vi "LINX - Live reset.vi"() -> ()   [LabVIEW 2019]
uses:
  <vilib>/MakerHub/LINX/Public/Utilities/Open Serial.vi
  <vilib>/MakerHub/LINX/LMH-LINX.lvlib
  vi.lib/LINXx/LINXx.lvlib
panel:
  out "Connected?":bool
  in  "Reconnect wait time":u32=2000
  out "Loop Rate (Hz)":u32
  in  "stop":bool
  in  "Serial Port":refnum<visa-resource-name>="N/A"
  in  "Reset board":bool
  # "Setup"
  # "Status"
  # "Commands"
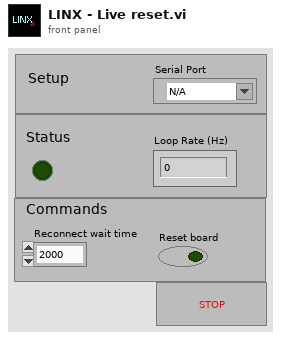
[diagram p1: front panel]
types:
  T1 = typedef "LMH-LINX.lvlib/LINX Ref.ctl" = cluster{"IO":T2, "Interface":T3, "LINX Device Config":T4}
  T2 = typedef "LMH-LINX.lvlib/Platform.ctl" = enum16{"Remote", "Local"}
  T3 = typedef "LMH-LINX.lvlib/Interface.ctl" = enum16{"Serial", "TCP"}
  T4 = typedef "LMH-LINX.lvlib/Device.lvlib/LINX Device Config.ctl" = cluster{"Interface":T3, "COM Port":refnum<visa-resource-name>, "TCP Configuration":T5, "Device Family":u8, "Device ID":u8, "Device Name":string, "TCP Ref":refnum<k5>, "Channels":T6}
  T5 = typedef "LMH-LINX.lvlib/Device.lvlib/TCP Config.ctl" = cluster{"IP Address":string, "Port":u16}
  T6 = typedef "LMH-LINX.lvlib/Channels.ctl" = cluster{"DI":u8[], "DO":u8[], "AI":u8[], "AO":u8[], "PWM":u8[], "QE":u8[], "UART":u8[], "I2C 2":u8[], "SPI":u8[], "CAN":u8[], "Servo":u8[], "AI Ref (V)":dbl, "AI Resolution (Bits)":u8, "AO Ref (V)":dbl, "AO Resolution (Bits)":u8}
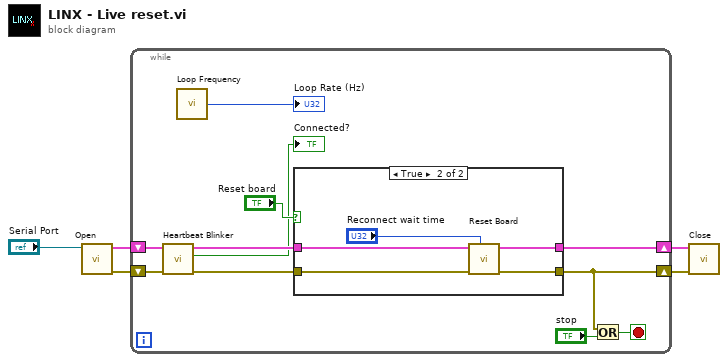
[diagram p0: block diagram]
diagram:
  n1 = call-poly <vilib>:"Open.vi"("Serial Port"="Serial Port") -> ("Error Out"=w4:errorcluster, "LINX Resource"=w5:T1)  [unwired: 8 in, 1 out]
  n2 = while {
    shift-right: [w15] -> w3
    shift-left: w5 -> [w8]
    shift-right: [w12] -> w2
    shift-left: w4 -> [w10]
    stop <- w13 stop-if-true
    n3 = call "Heartbeat Blinker.vi"("Error In"=w10, "LINX Resource"=w8) -> ("Error Out"=w9:errorcluster, "LED"=→"Connected?":bool, "LINX Resource Out"=w7:T1)  [unwired: 7 in]
    n4 = call <vilib>:"Loop Frequency.vi"() -> ("Loop Rate (Hz)"=→"Loop Rate (Hz)":u32)
    n5 = case shown="True" "Reset board" {
      tunnel: w7 -> [w18 w21]
      tunnel: [w18 w20] -> w15
      tunnel: [w17 w22] -> w12
      tunnel: w9 -> [w17 w23]
      frame False {
      }
      frame True {
        n6 = call "Reset Board.vi"("Reconnect wait time"="Reconnect wait time", "Error In"=w23, "LINX Resource"=w21) -> ("Error Out"=w22:errorcluster, "LINX Resource out"=w20:T1)  [unwired: 7 in]
      }
    }
    n7 = Or(x=w12, y="stop") -> (x .or. y?=w13:bool)
  }
  n8 = call <vilib>:"Close.vi"("Error In"=w2, "LINX Resource"=w3) -> ()  [unwired: 9 in, 1 out]
